vi "Send Packet.vi"(1 "Set":T1={"Filter Type"=0, "Baud-rate"=0, "Output Rate"=0, "Cutoff Frequency"=0, "Receiving ID"=100, "Transmitting ID First "=1, "Transmitting ID Second"=2} {"Cutoff Frequency" items=["No filtering", "500Hz", "300Hz", "200Hz", "150Hz", "100Hz", "50Hz", "40Hz", "30Hz", "20Hz", "10Hz", "5Hz", "3Hz"]; "Output Rate" items=["200Hz", "10Hz", "20Hz", "50Hz", "100Hz", "200Hz", "333Hz", "500Hz", "1000Hz"]; "Baud-rate" items=["115,200", "921,600", "460,800", "230,400", "115,200", "57,600"]; "Filter Type" items=["None", "LowPass Filter"]}, 2 "Command":u16(ring)=11 items=["Read Model Name", "Read S/N", "Read Firmware Ver.", "Set Communication ID", "Read Communication ID", "Set Baud-rate", "Read Baud-rate", "Set Filter", "Read Filter Setting", "F/T 1 sample Output", "F/T Output", "F/T Output Stop", "Reserved", "Reserved", "Set Output Rate", "Read Output Rate", "Bias Setting", "Read Overload log"]) -> (0 "Packet":u8[](array[numeric]))   [LabVIEW 2011]
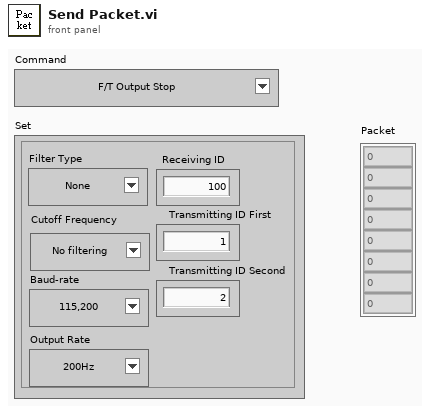
[diagram p1: front panel]
types:
  T1 = cluster{"Filter Type":u16, "Baud-rate":u16, "Output Rate":u16, "Cutoff Frequency":u8, "Receiving ID":u8, "Transmitting ID First ":u8, "Transmitting ID Second":u8}
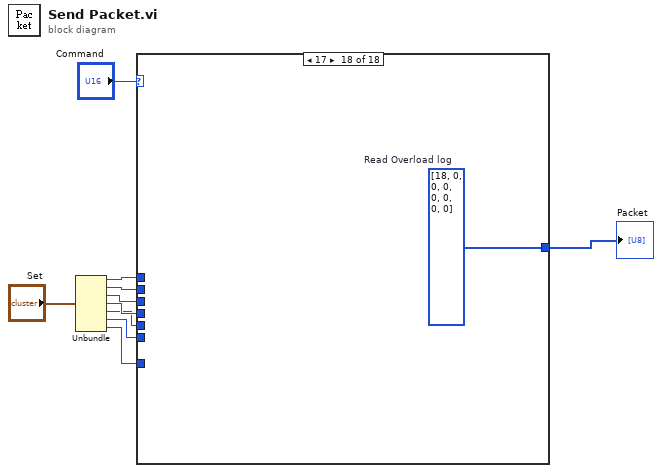
[diagram p0: block diagram]
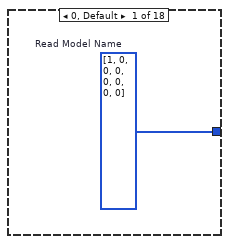
[diagram p2: hidden frame]
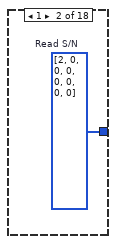
[diagram p3: hidden frame]
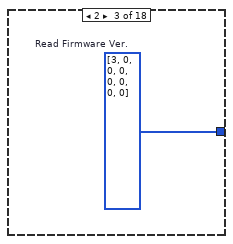
[diagram p4: hidden frame]
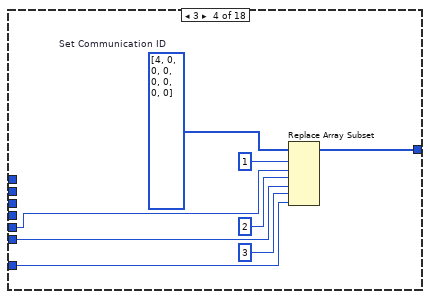
[diagram p5: hidden frame]
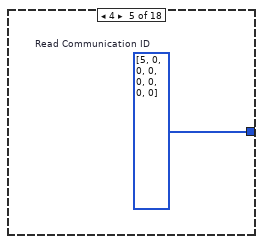
[diagram p6: hidden frame]
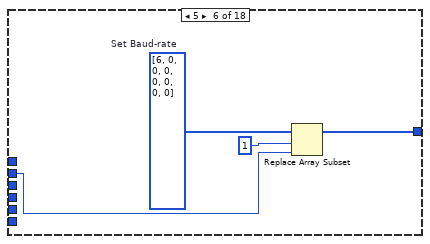
[diagram p7: hidden frame]
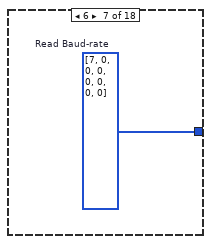
[diagram p8: hidden frame]
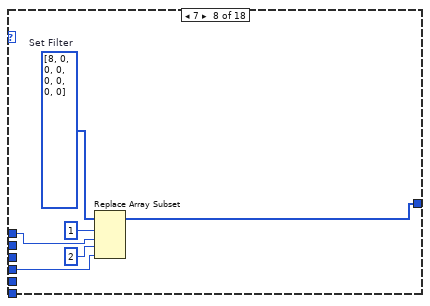
[diagram p9: hidden frame]
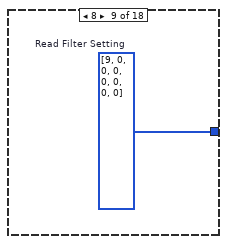
[diagram p10: hidden frame]
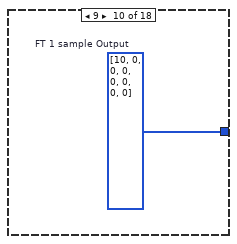
[diagram p11: hidden frame]
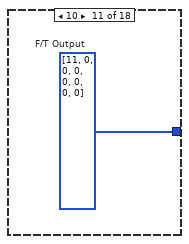
[diagram p12: hidden frame]
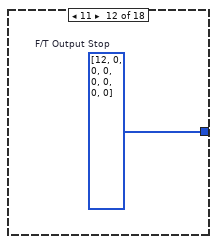
[diagram p13: hidden frame]
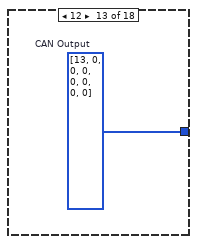
[diagram p14: hidden frame]
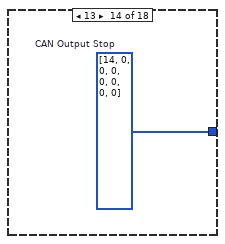
[diagram p15: hidden frame]
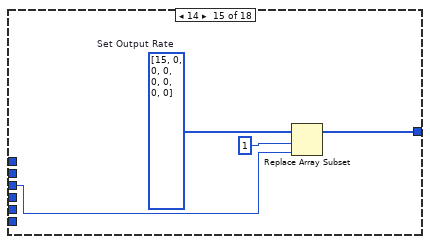
[diagram p16: hidden frame]
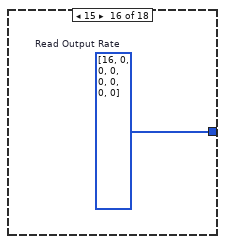
[diagram p17: hidden frame]
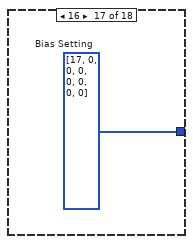
[diagram p18: hidden frame]
diagram:
  n1 = Unbundle("Set") -> ("Filter Type"=w7:u16, "Baud-rate"=w8:u16, "Output Rate"=w5:u16, "Cutoff Frequency"=w6:u8, "Receiving ID"=w3:u8, "Transmitting ID First"=w2:u8, "Transmitting ID Second"=w1:u8)
  n2 = case shown="17" "Command" {
    tunnel: [w11 w12 w13 w14 w22 w24 w27 w30 w34 w35 w36 w37 w38 w39 w41 w44 w45 w46] -> w10
    tunnel: w8 -> [_ _ _ _ _ w23 _ _ _ _ _ _ _ _ _ _ _ _]
    tunnel: w7 -> [_ _ _ _ _ _ _ w29 _ _ _ _ _ _ _ _ _ _]
    tunnel: w6 -> [_ _ _ _ _ _ _ w28 _ _ _ _ _ _ _ _ _ _]
    tunnel: w5 -> [_ _ _ _ _ _ _ _ _ _ _ _ _ _ w40 _ _ _]
    tunnel: w3 -> [_ _ _ w17 _ _ _ _ _ _ _ _ _ _ _ _ _ _]
    tunnel: w2 -> [_ _ _ w16 _ _ _ _ _ _ _ _ _ _ _ _ _ _]
    tunnel: w1 -> [_ _ _ w15 _ _ _ _ _ _ _ _ _ _ _ _ _ _]
    frame 0, Default {
      w11 = u8[] [1, 0, 0, 0, 0, 0, 0, 0]  # Read Model Name
    }
    frame 1 {
      w12 = u8[] [2, 0, 0, 0, 0, 0, 0, 0]  # Read S/N
    }
    frame 2 {
      w13 = u8[] [3, 0, 0, 0, 0, 0, 0, 0]  # Read Firmware Ver.
    }
    frame 3 {
      w21 = u8[] [4, 0, 0, 0, 0, 0, 0, 0]  # Set Communication ID
      n3 = Replace Array Subset(array=w21, new element #1=w17, index #1=1 ("인덱스"), new element #2=w16, index #2=2 ("인덱스"), new element #3=w15, index #3=3 ("인덱스")) -> (w14:u8[])
    }
    frame 4 {
      w22 = u8[] [5, 0, 0, 0, 0, 0, 0, 0]  # Read Communication ID
    }
    frame 5 {
      w25 = u8[] [6, 0, 0, 0, 0, 0, 0, 0]  # Set Baud-rate
      n4 = Replace Array Subset(array=w25, new element=w23, index=1 ("인덱스")) -> (w24:u8[])
    }
    frame 6 {
      w27 = u8[] [7, 0, 0, 0, 0, 0, 0, 0]  # Read Baud-rate
    }
    frame 7 {
      w32 = u8[] [8, 0, 0, 0, 0, 0, 0, 0]  # Set Filter
      n5 = Replace Array Subset(array=w32, new element #1=w29, index #1=1 ("인덱스"), new element #2=w28, index #2=2 ("인덱스")) -> (w30:u8[])
    }
    frame 8 {
      w34 = u8[] [9, 0, 0, 0, 0, 0, 0, 0]  # Read Filter Setting
    }
    frame 9 {
      w35 = u8[] [10, 0, 0, 0, 0, 0, 0, 0]  # FT 1 sample Output
    }
    frame 10 {
      w36 = u8[] [11, 0, 0, 0, 0, 0, 0, 0]  # F/T Output
    }
    frame 11 {
      w37 = u8[] [12, 0, 0, 0, 0, 0, 0, 0]  # F/T Output Stop
    }
    frame 12 {
      w38 = u8[] [13, 0, 0, 0, 0, 0, 0, 0]  # CAN Output
    }
    frame 13 {
      w39 = u8[] [14, 0, 0, 0, 0, 0, 0, 0]  # CAN Output Stop
    }
    frame 14 {
      w43 = u8[] [15, 0, 0, 0, 0, 0, 0, 0]  # Set Output Rate
      n6 = Replace Array Subset(array=w43, new element=w40, index=1 ("인덱스")) -> (w41:u8[])
    }
    frame 15 {
      w44 = u8[] [16, 0, 0, 0, 0, 0, 0, 0]  # Read Output Rate
    }
    frame 16 {
      w45 = u8[] [17, 0, 0, 0, 0, 0, 0, 0]  # Bias Setting
    }
    frame 17 {
      w46 = u8[] [18, 0, 0, 0, 0, 0, 0, 0]  # Read Overload log
    }
  }
  "Packet" <- w10
